vi "ni579x Construct Command Set Clock Phase DAC.vi"(0 "Register Bus":refnum<class "ni579x Register Bus v1 Host.lvclass">=refnum, 1 "scope":string, 5 "clock phase DAC value":u16, 11 "Error In":errorcluster) -> (4 "Register Bus (out)":refnum<class "ni579x Register Bus v1 Host.lvclass">, 6 "FAM Register Operations":T1[](array[typedef]) {"Write Data" format="%x"; "Address" format="%06x"; "FAM Register Offset" items=["ADC"=1, "DAC"=2, "Clock Distribution Chip"=3, "Frequency/Phase Adjust DAC"=4, "EEPROM"=5, "EEPROM Commands"=6, "LO1"=7, "Rx Atten Pre-LNA"=9, "Rx Atten Post-LNA"=10, "Tx Atten"=11]}, 10 "coerced clock phase DAC value":u16, 15 "Error Out":errorcluster)   [LabVIEW 2013]
uses:
  <instrlib>/ni579x/Register Bus/v1/Host/ni579x Register Bus v1 Host.lvclass
  <instrlib>/ni579x/Config/v1/Shared/Types/ni579x FAM Register Operation.ctl
  <instrlib>/ni579x/Config/v1/Shared/Types/ni579x FAM Register Offset.ctl
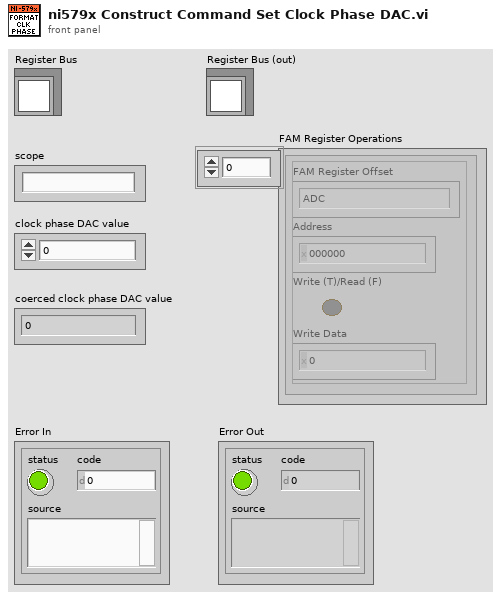
[diagram p1: front panel]
types:
  T1 = typedef "ni579x FAM Register Operation.ctl" = cluster{"FAM Register Offset":T2, "Address":u32, "Write (T)/Read (F)":bool, "Write Data":u32}
  T2 = typedef "ni579x FAM Register Offset.ctl" = u8
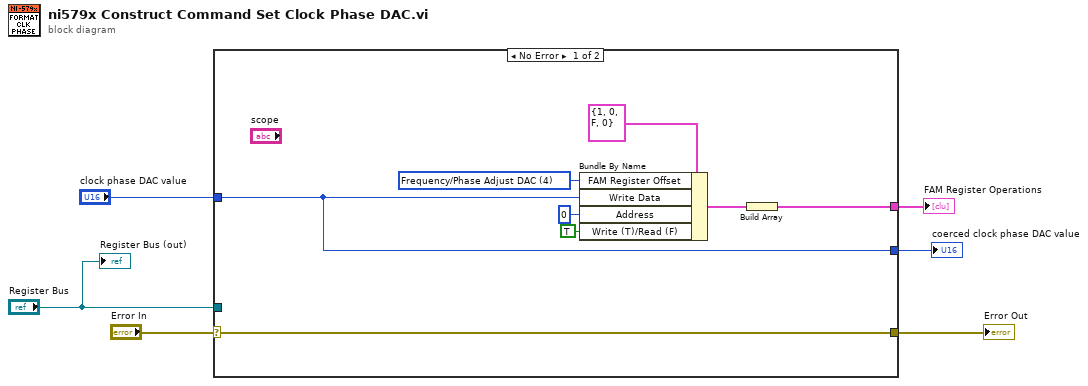
[diagram p0: block diagram]
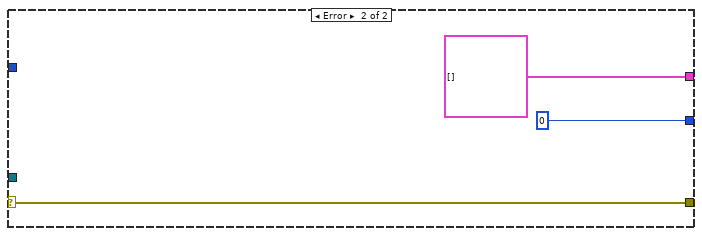
[diagram p2: hidden frame]
diagram:
  n1 = case shown="No Error" "Error In" {
    selector: "Error In" -> [w10 w17]
    tunnel: [w10 w17] -> w5
    tunnel: "Register Bus" -> [_ _]
    tunnel: [w8 T1[] [] ("SPI Instructions")] -> w3
    tunnel: "clock phase DAC value" -> [w7 _]
    tunnel: [w7 u16 0 ("clock phase DAC value")] -> w1
    frame No Error {
      w12 = T2 4 items=["ADC"=1, "DAC"=2, "Clock Distribution Chip"=3, "Frequency/Phase Adjust DAC"=4, "EEPROM"=5, "EEPROM Commands"=6, "LO1"=7, "Rx Atten Pre-LNA"=9, "Rx Atten Post-LNA"=10, "Tx Atten"=11] ("FAM Register Offset")
      n2 = Bundle By Name(cluster=T1 {"FAM Register Offset"=1, "Address"=0, "Write (T)/Read (F)"=FALSE, "Write Data"=0} ("FAM Register Operation"), "FAM Register Offset"=w12, "Write Data"=w7, "Address"=u32 0, "Write (T)/Read (F)"=TRUE) -> (w9:T1)
      n3 = Build Array(w9) -> (w8:T1[])
    }
    frame Error {
    }
  }
  "Error Out" <- w5
  "FAM Register Operations" <- w3
  "coerced clock phase DAC value" <- w1
  "Register Bus (out)" <- "Register Bus"
